vi "TestCaseInfoChange.vi"(3 "TestCaseInfo":string[](array[string])=["project", "subfolder", "filename", "measurementnumber"]) -> (1 "JSON Tree out (JSON Object)":variant)   [LabVIEW 2018]
uses:
  <vilib>/LVH/i3 JSON/JSON Generation/Create Value Files/Create Value - Object.vi
  <vilib>/LVH/i3 JSON/JSON Generation/Add Object Parameter Files/Add Object Parameter - String.vi
  <vilib>/LVH/i3 JSON/JSON Generation/Add Object Parameter Files/Add Object Parameter - Object.vi
  <vilib>/LVH/i3 JSON/i3-json.lvlib
panel:
  out "String":string
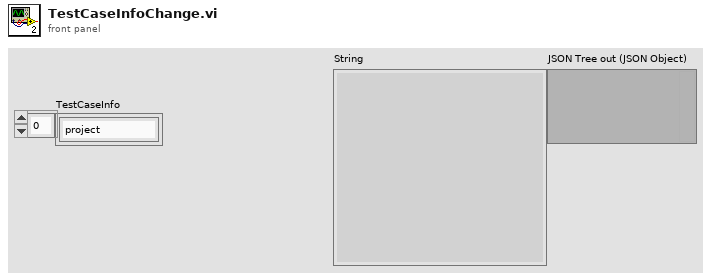
[diagram p1: front panel]
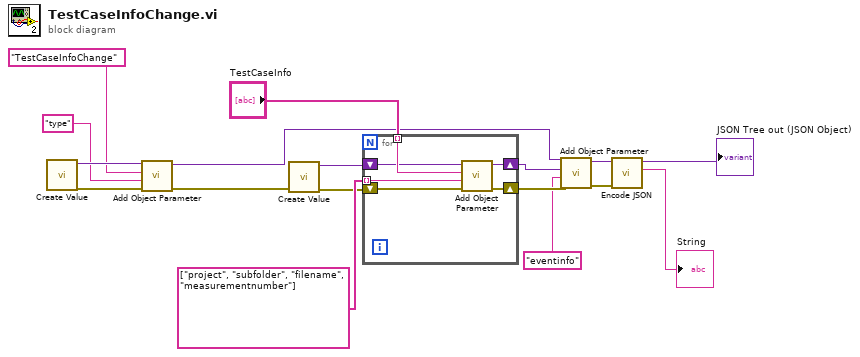
[diagram p0: block diagram]
diagram:
  n1 = call-poly <vilib>:"Create Value.vi"() -> ("error out"=w13:errorcluster, "JSON Tree"=w14:variant)  [unwired: 10 in]
  n2 = call-poly <vilib>:"Add Object Parameter.vi"("error in (no error)"=w13, "Name"="type", "String"="TestCaseInfoChange", "JSON Tree in (JSON Object)"=w14) -> ("error out"=w10:errorcluster, "JSON Tree out (JSON Object)"=w8:variant)  [unwired: 6 in]
  n3 = call-poly <vilib>:"Create Value.vi"("error in (no error)"=w10) -> ("error out"=w9:errorcluster, "JSON Tree"=w5:variant)  [unwired: 9 in]
  n4 = for {
    tunnel: string[] ["project", "subfolder", "filename", "measurementnumber"] -> [w22] mode=indexing
    tunnel: "TestCaseInfo" -> [w21] mode=indexing
    shift-right: [w18] -> w7
    shift-left: w9 -> [w20]
    shift-right: [w19] -> w6
    shift-left: w5 -> [w17]
    n5 = call-poly <vilib>:"Add Object Parameter.vi"("error in (no error)"=w20, "Name"=w22, "String"=w21, "JSON Tree in (JSON Object)"=w17) -> ("error out"=w18:errorcluster, "JSON Tree out (JSON Object)"=w19:variant)  [unwired: 6 in]
  }
  n6 = call-poly <vilib>:"Add Object Parameter.vi"("error in (no error)"=w7, "Name"="eventinfo", "JSON Object"=w6, "JSON Tree in (JSON Object)"=w8) -> ("error out"=w3:errorcluster, "JSON Tree out (JSON Object)"=w2:variant)  [unwired: 6 in]
  "JSON Tree out (JSON Object)" <- w2
  n7 = call <vilib>:"Encode JSON.vi"("error in (no error)"=w3, "JSON Tree"=w2) -> ("String"=→"String":string)  [unwired: 4 in, 1 out]
